vi "Update-processing-variables.vi"(8 "error in (no error)":errorcluster, 11 "Data ref. in":refnum<data-value>) -> (0 "error out":errorcluster, 3 "Data ref.":refnum<data-value>)   [LabVIEW 2013, in "CameraVision.lvlib" / "CV-Main.lvclass"]
uses:
  CV-Main.lvclass
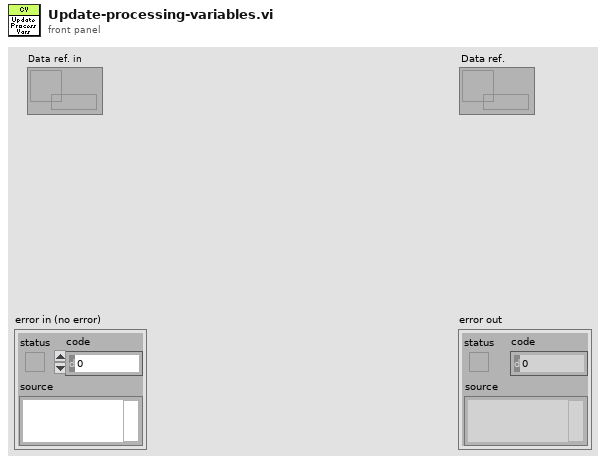
[diagram p1: front panel]
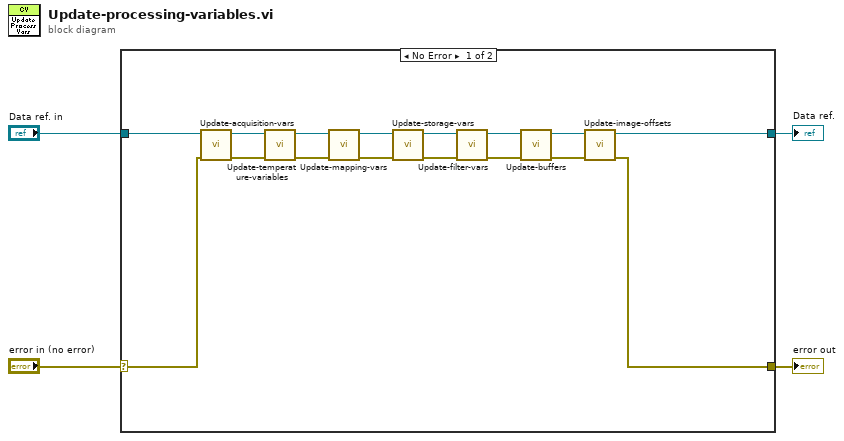
[diagram p0: block diagram]
diagram:
  n1 = case shown="No Error" "error in (no error)" {
    selector: "error in (no error)" -> [w7 w22]
    tunnel: [w10 w22] -> w3
    tunnel: "Data ref. in" -> [w6 w21]
    tunnel: [w9 w21] -> w1
    frame No Error {
      n2 = call "Update-acquisition-vars.vi"("error in"=w7, "Data ref. in"=w6) -> ("error IO"=w8:errorcluster, "Data ref."=w5:refnum<data-value>)  [unwired: 6 in, 2 out]
      n3 = call "Update-temperature-variables.vi"("error in"=w8, "Data ref. in"=w5) -> ("error IO"=w20:errorcluster, "Data ref."=w17:refnum<data-value>)  [unwired: 8 in]
      n4 = call "Update-mapping-vars.vi"("error in"=w20, "Data ref. in"=w17) -> ("error IO"=w19:errorcluster, "Data ref."=w16:refnum<data-value>)  [unwired: 8 in]
      n5 = call "Update-storage-vars.vi"("error in"=w19, "Data ref. in"=w16) -> ("error IO"=w18:errorcluster, "Data ref."=w15:refnum<data-value>)  [unwired: 8 in]
      n6 = call "Update-filter-vars.vi"("error in"=w18, "Data ref. in"=w15) -> ("error IO"=w14:errorcluster, "Data ref."=w13:refnum<data-value>)  [unwired: 8 in]
      n7 = call "Update-buffers.vi"("error in"=w14, "Data ref. in"=w13) -> ("error IO"=w12:errorcluster, "Data ref."=w11:refnum<data-value>)  [unwired: 8 in]
      n8 = call "Update-image-offsets.vi"("error in (no error)"=w12, "Data ref. in"=w11) -> ("error out"=w10:errorcluster, "Data ref."=w9:refnum<data-value>)  [unwired: 5 in, 3 out]
    }
    frame Error {
    }
  }
  "error out" <- w3
  "Data ref." <- w1
